vi "F2Imageglobal.vi"(4 "max":sgl format="%.2f", 5 "Palette Number (gray)":T2(ring), 6 "min":sgl format="%.2f", 8 "error in":errorcluster, 9 "Fx channel":u8, 10 "input Image array":u8[][](array[numeric]), 11 "Enum":T1(ring)) -> (0 "error out":errorcluster, 1 "String":string, 3 "New Image":T3)   [LabVIEW 2009]
uses:
  <vilib>/vision/Image Controls.llb/IMAQ Image.ctl
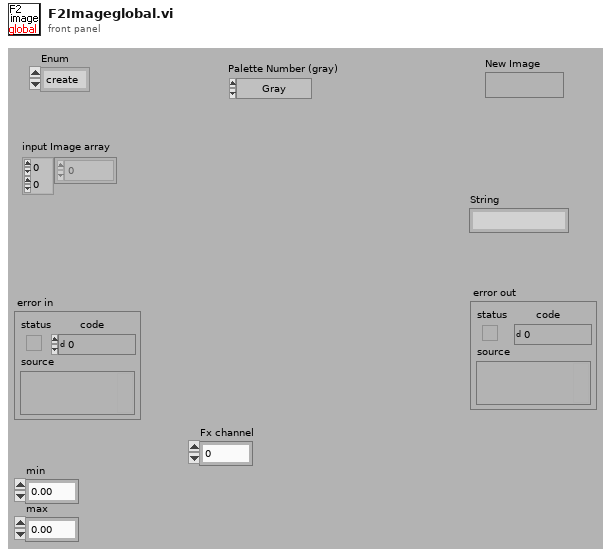
[diagram p1: front panel]
types:
  T1 = enum16{"create", "Input", "draw", "colorpal", "dump", "Get", "kill"}
  T2 = enum32{"Gray", "Binary", "Gradient", "Rainbow", "Temperature"}
  T3 = typedef "IMAQ Image.ctl" = refnum<image>
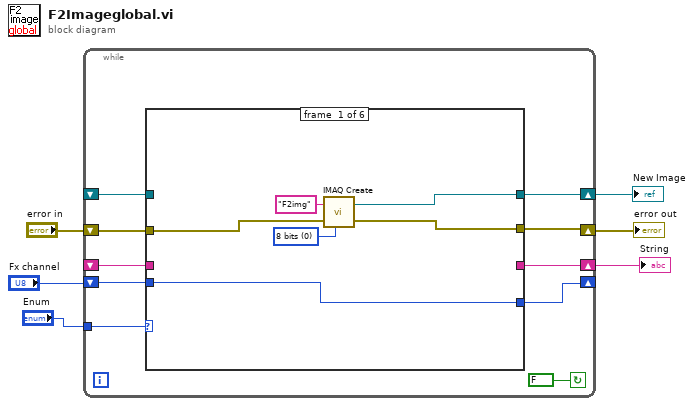
[diagram p0: block diagram]
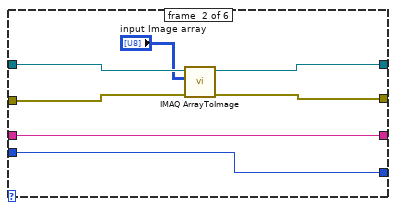
[diagram p2: hidden frame]
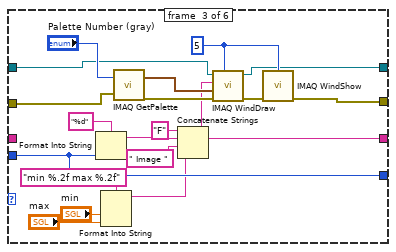
[diagram p3: hidden frame]
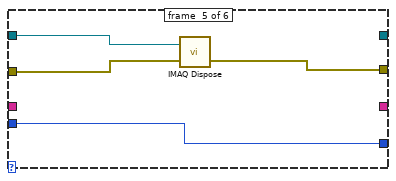
[diagram p5: hidden frame]
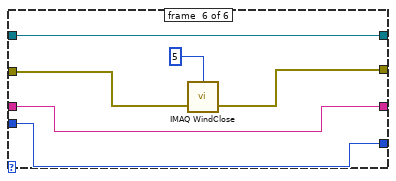
[diagram p6: hidden frame]
diagram:
  n1 = while {
    shift-right: [w14] -> w6
    shift-left: _ -> [w16]
    shift-right: [w13] -> w5
    shift-left: "error in" -> [w15]
    shift-right: [w12] -> w3
    shift-left: _ -> [w11]
    shift-right: [w9] -> _
    shift-left: "Fx channel" -> [w10]
    tunnel: "Enum" -> [w8]
    stop <- FALSE continue-if-true
    n2 = case shown="\"kill\"" w8 {
      tunnel: w16 -> [_ w27 w44 w51 w55 w57]
      tunnel: w15 -> [w19 w29 w48 _ w54 w61]
      tunnel: [w20 w26 w40 w51 _ w57] -> w14
      tunnel: [w18 w28 w42 _ w53 w60] -> w13
      tunnel: [_ w24 w37 w50 _ w58] -> w12
      tunnel: w11 -> [_ w24 _ w50 _ w58]
      tunnel: w10 -> [w17 w23 w34 w49 w52 w56]
      tunnel: [w17 w23 w34 w49 w52 w56] -> w9
      frame #0 {
        w21 = u32 0 items=["8 bits", "16 bits", "Float", "Complex", "RGB", "HSL"] ("Image Type")
        n3 = call "IMAQ Create"("Image Name"="F2img", "Image Type"=w21, "error in (no error)"=w19) -> ("New Image"=w20:T3, "error out"=w18:errorcluster)  [unwired: 2 in]
      }
      frame #1 {
        n4 = call "IMAQ ArrayToImage"("error in (no error)"=w29, "Image Pixels (U8)"="input Image array", "Image"=w27) -> ("error out"=w28:errorcluster, "Image Out"=w26:T3)  [unwired: 7 in]
      }
      frame #2 {
        w41 = 5 ("Window Number (0...15)")
        n5 = Format Into String(format string="%d", w34) -> (resulting string=w36:string)  [unwired: 2 in, 1 out]
        n6 = Format Into String(format string="min %.2f max %.2f", "min", "max") -> (resulting string=w30:string)  [unwired: 2 in, 1 out]
        n7 = call "IMAQ GetPalette"("Palette Number (gray)"="Palette Number (gray)", "error in (no error)"=w48) -> ("Color Palette"=w45:cluster{"Red":u8, "Green":u8, "Blue":u8}[], "error out"=w46:errorcluster)  [unwired: 3 in]
        n8 = Concatenate Strings("F" ("string"), w36, " Image " ("string"), w30) -> (w37:string)
        n9 = call "IMAQ WindDraw"("Window Number (0...15)"=w41, "error in (no error)"=w46, "Color Palette"=w45, "Title"=w37, "Image"=w44) -> ("error out"=w43:errorcluster, "Image Out (duplicate)"=w40:T3)  [unwired: 5 in]
        n10 = call "IMAQ WindShow"("error in (no error)"=w43, "Window Number (0...15)"=w41) -> ("error out"=w42:errorcluster)  [unwired: 4 in, 2 out]
      }
      frame #3 {
      }
      frame #4 {
        n11 = call "IMAQ Dispose"("Image"=w55, "error in (no error)"=w54) -> ("error out"=w53:errorcluster)  [unwired: 4 in]
      }
      frame #5 {
        n12 = call "IMAQ WindClose"("Window Number (0...15)"=5, "error in (no error)"=w61) -> ("error out"=w60:errorcluster)  [unwired: 4 in]
      }
    }
  }
  "New Image" <- w6
  "error out" <- w5
  "String" <- w3
